vi "Periodic Tasks.vi"(8 "error in":errorcluster) -> ()   [LabVIEW 2016]
doc: "This VI runs in parallel to other tasks. It can contain as many user-defined periodic loops as you need. These can carry out PID or other sorts of timed response."
uses:
  Robot Global Data.vi
  <vilib>/Rock Robotics/Network Tables/NT Write Number.vi
panel:
  out "Heading":dbl
  out "Sonic":dbl
  out "RollerSw":bool
  out "GearSw":bool
  out "RDist":dbl
  out "LDist":dbl
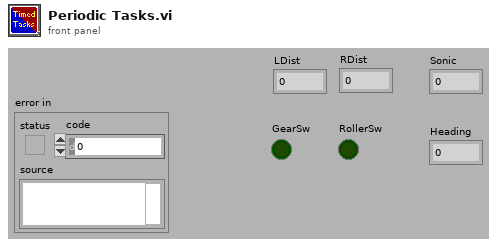
[diagram p1: front panel]
types:
  T1 = typedef "WPI_SwitchDevRef.ctl" = cluster{"DevStatus":errorcluster, "DIO Channel":T2, "CntIndex":T3, "Normally Closed":bool}
  T2 = typedef "FPGA_DIOChannel.ctl" = enum8{"DIO 0", "DIO 1", "DIO 2", "DIO 3", "DIO 4", "DIO 5", "DIO 6", "DIO 7", "DIO 8", "DIO 9", "DIO MXP 0", "DIO MXP 1", "DIO MXP 2", "DIO MXP 3", "DIO MXP 4", "DIO MXP 5", "DIO MXP 6", "DIO MXP 7", "DIO MXP 8", "DIO MXP 9", "DIO MXP 10", "DIO MXP 11", "DIO MXP 12", "DIO MXP 13", "DIO MXP 14", "DIO MXP 15", "SPI Port CS1", "SPI Port CS2", "SPI Port CS3", "SPI Port MISO", "SPI Port MOSI", "Invalid"}
  T3 = typedef "FPGA_CounterCtrSystemIndex.ctl" = enum8{"Ctr 0", "Ctr 1", "Ctr 2", "Ctr 3", "Ctr 4", "Ctr 5", "Ctr 6", "Ctr 7", "Invalid"}
  T4 = typedef "WPI_CounterDevRef.ctl" = cluster{"DevStatus":errorcluster, "CntIndex":T3}
  T5 = typedef "WPI_EncoderDevRef.ctl" = cluster{"DevStatus":errorcluster, "EncoderIndex":T6, "CounterIndex":T3, "DistancePerCount":dbl, "Decoding Type":T7}
  T6 = typedef "FPGA_EncoderIdx.ctl" = enum8{"Enc 0", "Enc 1", "Enc 2", "Enc 3", "Enc 4", "Enc 5", "Enc 6", "Enc 7", "Invalid"}
  T7 = typedef "WPI_EncoderType.ctl" = enum16{"1x", "2x", "4x"}
  T8 = typedef "WPI_GyroDevRef.ctl" = cluster{"DevStatus":errorcluster, "Analog Channel":T9, "Offset":dbl, "Gain (VoltsPerDegree/Second)":dbl, "Gyro Type":enum16{"Analog", "XRS450"}, "Handle":i32, "SPI Bus":T10, "Device Found":bool, "Sample Rate":dbl, "Calibrate On Open":bool}
  T9 = typedef "FPGA_AIChannel.ctl" = enum8{"AI 0", "AI 1", "AI 2", "AI 3", "AI MXP 0", "AI MXP 1", "AI MXP 2", "AI MXP 3", "Invalid"}
  T10 = typedef "spi_bus.ctl" = enum16{"SPI On-Board, CS0", "SPI On-Board, CS1", "SPI On-Board, CS2", "SPI On-Board, CS3", "SPI MXP", "Invalid"}
  T11 = typedef "WPI_MotorControlDeviceRef.ctl" = cluster{"DeviceStatus":errorcluster, "Type":T12, "PWM":cluster{"PWM Channel":T13, "DeadBand":T14}, "CAN":cluster{"Device Number":u8, "SetOutput VI Ref":variant, "GetOutput VI Ref":variant, "Enable VI Ref":variant, "Disable VI Ref":variant, "Data":variant}, "Invert":bool}
  T12 = typedef "WPI_MotorControlType.ctl" = enum16{"PWM", "CAN"}
  T13 = typedef "FPGA_DIOPWMChannel.ctl" = enum8{"PWM 0", "PWM 1", "PWM 2", "PWM 3", "PWM 4", "PWM 5", "PWM 6", "PWM 7", "PWM 8", "PWM 9", "PWM MXP 0", "PWM MXP 1", "PWM MXP 2", "PWM MXP 3", "PWM MXP 4", "PWM MXP 5", "PWM MXP 6", "PWM MXP 7", "PWM MXP 8", "PWM MXP 9", "Invalid"}
  T14 = typedef "WPI_PWMDeadband.ctl" = cluster{"Name":string, "maxPositivePwm":i32, "minPositivePwm":i32, "centerPwm":i32, "maxNegativePwm":i32, "minNegativePwm":i32, "angularRange":u16}
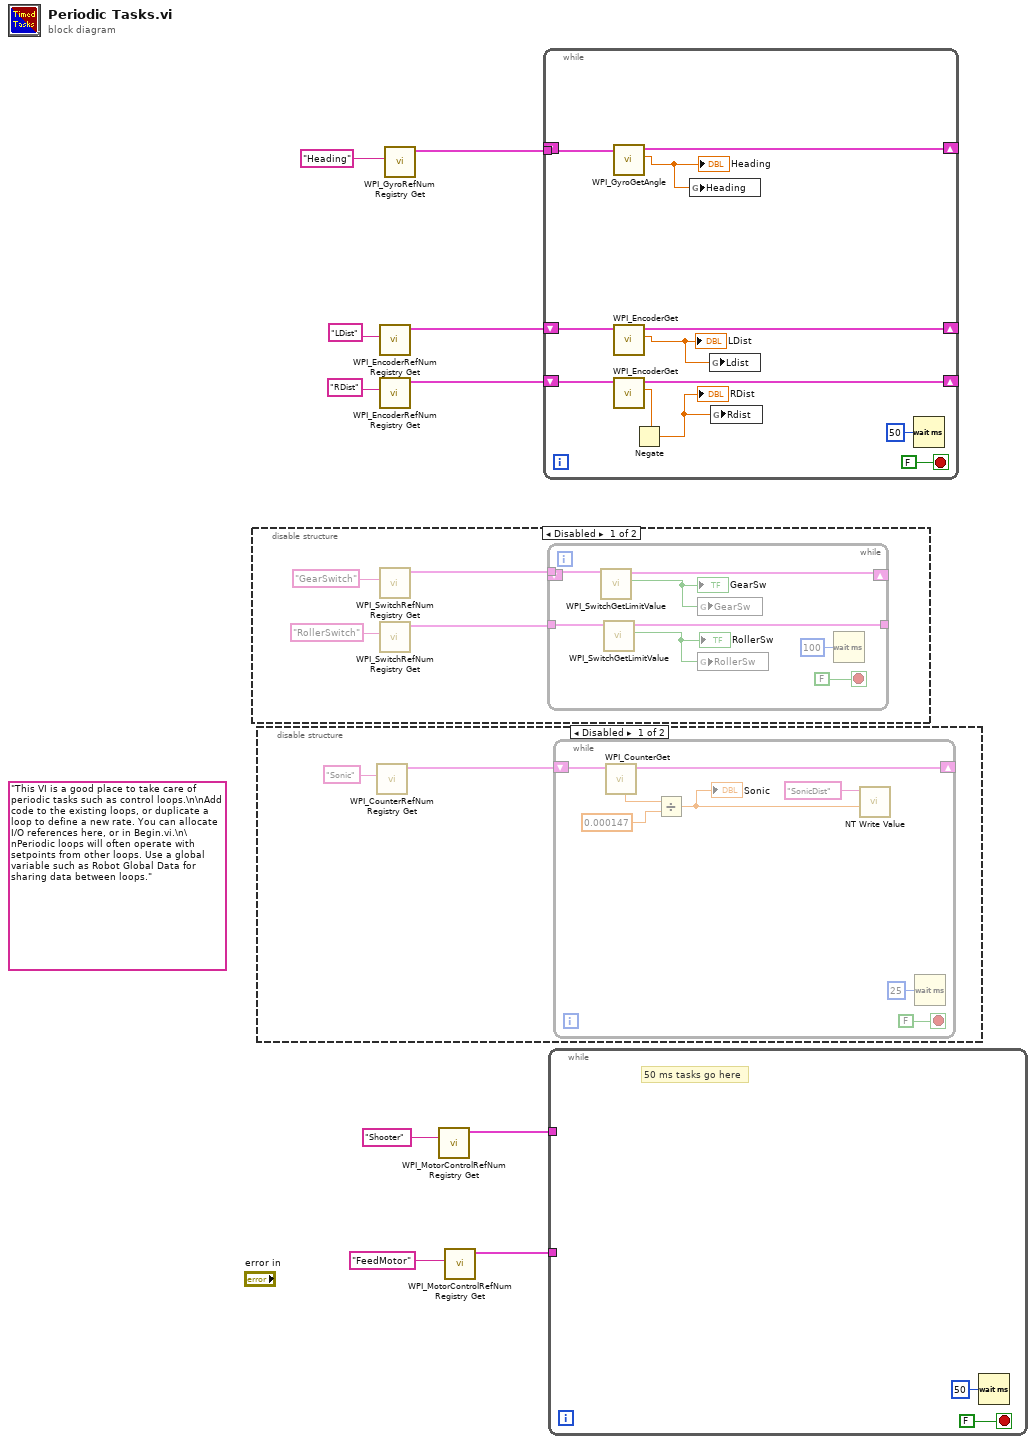
[diagram p0: block diagram]
diagram:
  (unwired) "This VI is a good place to take care of periodic tasks such as control loops.\n\nAdd code to the existing loops, or duplicate a loop to define a new rate. You can allocate I/O references here, or in Begin.vi.\n\nPeriodic loops will often operate with setpoints from other loops. Use a global variable such as Robot Global Data for sharing data between loops."
  n1 = disable-structure shown="Disabled" {
    frame Disabled {
      n2 = call <vilib>:"WPI_SwitchRefNum Registry Get.vi"("refnum name"="GearSwitch") -> ("SwitchDevRef"=w12:T1)  [unwired: 9 in, 1 out]
      n3 = call <vilib>:"WPI_SwitchRefNum Registry Get.vi"("refnum name"="RollerSwitch") -> ("SwitchDevRef"=w11:T1)  [unwired: 9 in, 1 out]
      n4 = while {
        tunnel: w12 -> [w20]
        shift-right: [w19] -> _
        shift-left: _ -> [_]
        tunnel: w11 -> [w16]
        tunnel: [w15] -> _
        stop <- FALSE stop-if-true
        n5 = call <vilib>:"WPI_SwitchGetLimitValue.vi"("SwitchDevRef"=w20) -> ("Switch Pressed"=w18:bool, "SwitchDevRef"=w19:T1)  [unwired: 8 in, 1 out]
        "GearSw" <- w18
        n6 = call <vilib>:"WPI_SwitchGetLimitValue.vi"("SwitchDevRef"=w16) -> ("Switch Pressed"=w17:bool, "SwitchDevRef"=w15:T1)  [unwired: 8 in, 1 out]
        "RollerSw" <- w17
        n7 = global write "Robot Global Data.vi" "GearSw"(w18) -> ()
        n8 = global write "Robot Global Data.vi" "RollerSw"(w17) -> ()
        n9 = Wait (ms)(milliseconds to wait=u32 100) -> ()  [unwired: 1 out]
      }
    }
    frame Enabled {
    }
  }
  n10 = disable-structure shown="Disabled" {
    frame Disabled {
      n11 = call <vilib>:"WPI_CounterRefNum Registry Get.vi"("refnum name"="Sonic") -> ("CounterDevRef"=w23:T4)  [unwired: 9 in, 1 out]
      n12 = while {
        shift-right: [w27] -> _
        shift-left: w23 -> [w30]
        stop <- FALSE stop-if-true
        n13 = call <vilib>:"WPI_CounterGet.vi"("CounterDevRef in"=w30) -> ("CounterDevRef out"=w27:T4, "Period (sec)"=w29:dbl)  [unwired: 5 in, 4 out]
        n14 = Divide(x=w29, y=0.000147) -> (x/y=w25:dbl)
        "Sonic" <- w25
        n15 = call-poly <vilib>:"NT Write Value.vi"("Numeric"=w25, "Name"="SonicDist") -> ()  [unwired: 9 in, 1 out]
        n16 = Wait (ms)(milliseconds to wait=u32 25) -> ()  [unwired: 1 out]
      }
    }
    frame Enabled {
    }
  }
  n17 = call <vilib>:"WPI_EncoderRefNum Registry Get.vi"("refnum name"="LDist") -> ("EncoderDevRef"=w8:T5)  [unwired: 9 in, 1 out]
  n18 = call <vilib>:"WPI_EncoderRefNum Registry Get.vi"("refnum name"="RDist") -> ("EncoderDevRef"=w7:T5)  [unwired: 9 in, 1 out]
  n19 = call <vilib>:"WPI_GyroRefNum Registry Get.vi"("refnum name"="Heading") -> ("GyroDevRef"=w1:T8)  [unwired: 9 in, 1 out]
  n20 = call <vilib>:"WPI_MotorControlRefNum Registry Get.vi"("refnum name"="Shooter") -> ("MotorControlDevRef"=w4:T11)  [unwired: 9 in, 1 out]
  n21 = call <vilib>:"WPI_MotorControlRefNum Registry Get.vi"("refnum name"="FeedMotor") -> ("MotorControlDevRef"=w3:T11)  [unwired: 9 in, 1 out]
  n22 = while {
    shift-right: [w41] -> _
    shift-left: w8 -> [w42]
    shift-right: [w39] -> _
    shift-left: w7 -> [w40]
    tunnel: w1 -> [w37]
    shift-right: [w36] -> _
    shift-left: _ -> [_]
    stop <- FALSE stop-if-true
    n23 = call <vilib>:"WPI_GyroGetAngle.vi"("GyroDevRef"=w37) -> ("Angle"=w35:dbl, "GyroDevRef"=w36:T8)  [unwired: 6 in, 3 out]
    "Heading" <- w35
    n24 = call <vilib>:"WPI_EncoderGet.vi"("EncoderDevRef"=w42) -> ("Distance"=w38:dbl, "EncoderDevRef"=w41:T5)  [unwired: 5 in, 4 out]
    "LDist" <- w38
    n25 = call <vilib>:"WPI_EncoderGet.vi"("EncoderDevRef"=w40) -> ("Distance"=w34:dbl, "EncoderDevRef"=w39:T5)  [unwired: 5 in, 4 out]
    n26 = Negate(x=w34) -> (-x=w33:dbl)
    "RDist" <- w33
    n27 = global write "Robot Global Data.vi" "Heading"(w35) -> ()
    n28 = global write "Robot Global Data.vi" "Ldist"(w38) -> ()
    n29 = global write "Robot Global Data.vi" "Rdist"(w33) -> ()
    n30 = Wait (ms)(milliseconds to wait=u32 50) -> ()  [unwired: 1 out]
  }
  n31 = while {
    tunnel: w4 -> [_]
    tunnel: w3 -> [_]
    stop <- FALSE stop-if-true
    # "50 ms tasks go here"
    n32 = Wait (ms)(milliseconds to wait=u32 50) -> ()  [unwired: 1 out]
  }
